vi "Bairstow_ds&dr from P(x).vi"(9 "r":dbl, 10 "s":dbl, 11 "P(x)":dbl[](array[numeric])) -> (2 "dr":dbl, 3 "ds":dbl)   [LabVIEW 2018, in "NI_AALPro.lvlib"]
uses:
  NI_AALPro.lvlib
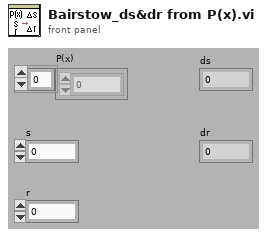
[diagram p1: front panel]
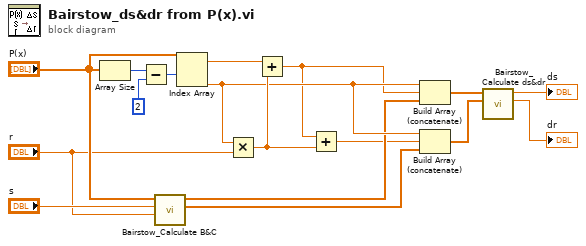
[diagram p0: block diagram]
diagram:
  n1 = Array Size(array="P(x)") -> (size(s)=w13:i32)
  n2 = Subtract(x=w13, y=2) -> (x-y=w15:i32)
  n3 = call "Bairstow_Calculate B&C.vi"("r"="r", "s"="s", "P(x)"="P(x)") -> ("C"=w2:dbl[], "B"=w3:dbl[])  [unwired: 7 in]
  n4 = Index Array(array="P(x)", index #1=w15) -> (element #1=w16:dbl, element #2=w5:dbl)  [unwired: 1 in]
  n5 = Multiply(x=w5, y="r") -> (x*y=w17:dbl)
  n6 = Add(x=w16, y=w17) -> (x+y=w4:dbl)
  n7 = Add(x=w4, y=w17) -> (x+y=w1:dbl)
  n8 = Build Array (concatenate)(w5, w4, w3) -> (w9:dbl[])
  n9 = Build Array (concatenate)(w5, w1, w2) -> (w8:dbl[])
  n10 = call "Bairstow_Calculate ds&dr.vi"("C"=w8, "B"=w9) -> ("dr"=→"dr":dbl, "ds"=→"ds":dbl)  [unwired: 8 in]
